vi "Process Player Weapon Inputs.vi"(11 "Ship in":refnum<class "Ship.lvclass">) -> (3 "Ship out":refnum<class "Ship.lvclass">)   [LabVIEW 2021, in "Ship.lvclass"]
uses:
  Ship.lvclass
  Ship.lvclass/Ship.ctl
  C:/dev/LabVIEW/LabMelee/Source/Application Specific/Element/Element.lvclass
  C:/dev/LabVIEW/LabMelee/Source/Application Specific/Ship/Ship.lvclass
  Control State/Control State.lvclass
  Element/Element.lvclass
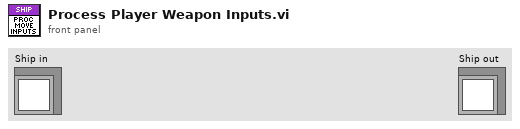
[diagram p1: front panel]
types:
  T1 = typedef "Control State.lvclass/Button State.ctl" = enum16{"Undefined", "Pressed", "Released", "Held", "Not Held"}
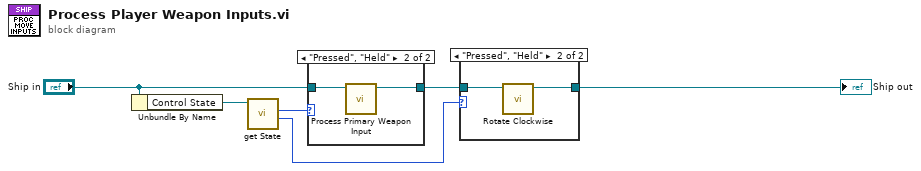
[diagram p0: block diagram]
diagram:
  n1 = Unbundle By Name("Ship in") -> ("Control State"=w4:refnum<class "Control State.lvclass">)
  n2 = call "get State.vi"("Control State in"=w4) -> ("Special Function"=w1:T1, "Primary Weapon"=w3:T1)  [unwired: 6 in, 3 out]
  n3 = case shown="\"Pressed\", \"Held\"" w3 {
    tunnel: "Ship in" -> [w7 w9]
    tunnel: [w7 w8] -> w6
    frame Default {
    }
    frame "Pressed", "Held" {
      n4 = call "Process Primary Weapon Input.vi"("Ship in"=w9) -> ("Ship out"=w8:refnum<class "Ship.lvclass">)  [unwired: 10 in]
    }
  }
  n5 = case shown="\"Pressed\", \"Held\"" w1 {
    tunnel: w6 -> [w10 w12]
    tunnel: [w10 w11] -> w2
    frame Default {
    }
    frame "Pressed", "Held" {
      n6 = call "Rotate Clockwise.vi"("Element in"=w12) -> ("Element out"=w11:refnum<class "Ship.lvclass">)  [unwired: 10 in]
    }
  }
  "Ship out" <- w2
